vi "LED Values.vi"() -> ()   [LabVIEW 2014]
panel:
  in  "LED Bits":u8[](array[numeric]) format="%.0x"
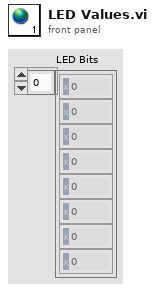
[diagram p1: front panel]
diagram:
